vi "Switch Select Instruments to Use.vi"(1 "Switch Type":T1=enum."Simulator", 3 "Instruments on Station":T2[](array[typedef])) -> (0 "SWI Instrument Record":T2)   [LabVIEW 2011]
uses:
  server/database/Stations/Instruments/Instrument Record.ctl
  TypeDefs/Switch Type.ctl
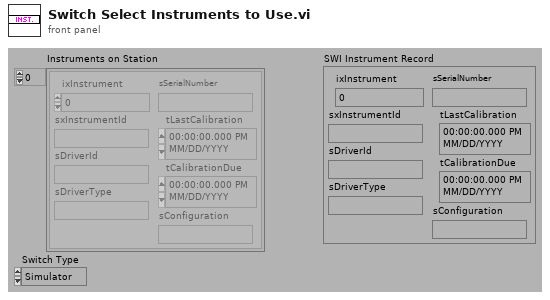
[diagram p1: front panel]
types:
  T1 = typedef "Switch Type.ctl" = enum16{"Sea-Level", "Simulator", "SI-0206-SW", "SI-0309-SW", "SI-0310-SW", "Front End"}
  T2 = typedef "Instrument Record.ctl" = cluster{"ixInstrument":i32, "sxInstrumentId":string, "sDriverId":string, "sDriverType":string, "sSerialNumber":string, "tLastCalibration":timestamp, "tCalibrationDue":timestamp, "sConfiguration":string}
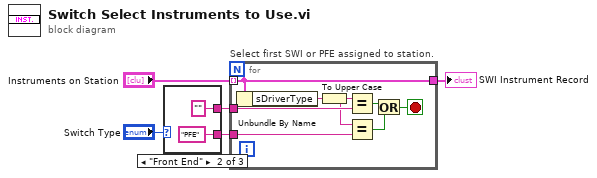
[diagram p0: block diagram]
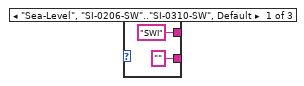
[diagram p2: hidden frame]
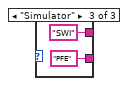
[diagram p3: hidden frame]
diagram:
  n1 = case shown="\"Front End\"" "Switch Type" {
    tunnel: ["SWI" ("y") "" ("y") "SWI" ("y")] -> w2
    tunnel: ["" ("y") "PFE" ("y") "PFE" ("y")] -> w1
    frame "Sea-Level", "SI-0206-SW".."SI-0310-SW", Default {
    }
    frame "Front End" {
    }
    frame "Simulator" {
    }
  }
  n2 = for "Select first SWI or PFE assigned to station." {
    tunnel: "Instruments on Station" -> [w18] mode=indexing
    tunnel: [w18] -> w4
    tunnel: w2 -> [w14]
    tunnel: w1 -> [w13]
    stop <- w16 stop-if-true
    n3 = Unbundle By Name(w18) -> ("sDriverType"=w19:string)
    n4 = To Upper Case(1:w19) -> (0:w12:string)
    n5 = Equal?(x=w12, y=w14) -> (x = y?=w17:bool)
    n6 = Equal?(x=w12, y=w13) -> (x = y?=w15:bool)
    n7 = Or(x=w17, y=w15) -> (x .or. y?=w16:bool)
  }
  "SWI Instrument Record" <- w4
